vi "Launch Instrumentstudio.vi"(11 "error in (no error)":errorcluster) -> (15 "error out":errorcluster)   [LabVIEW 2021, in "Converter.lvlib"]
uses:
  Converter.lvlib
  Path Functions/Path Functions.lvlib
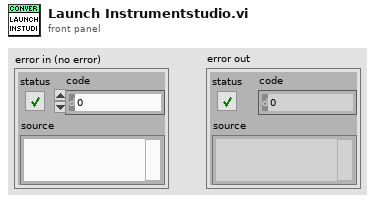
[diagram p1: front panel]
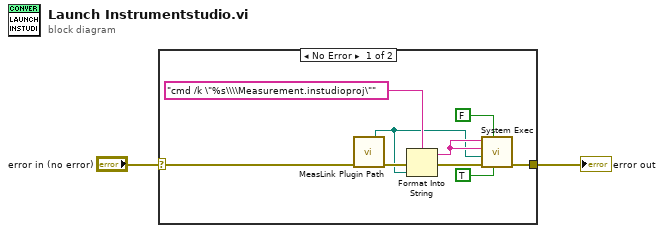
[diagram p0: block diagram]
diagram:
  n1 = case shown="No Error" "error in (no error)" {
    selector: "error in (no error)" -> [w9 w12]
    tunnel: [w3 w12] -> w1
    frame No Error {
      n2 = call "MeasLink Plugin Path.vi"("error in (no error)"=w9) -> ("Instrumentstudio Folder"=w5:path, "error out"=w10:errorcluster)  [unwired: 2 in, 11 out]
      n3 = Format Into String(format string="cmd /k \"%s\\\\Measurement.instudioproj\"", error in=w10, w5) -> (resulting string=w6:string, error out=w8:errorcluster)  [unwired: 1 in]
      n4 = call <vilib>:"System Exec.vi"("run minimized? (F)"=TRUE, "wait until completion? (T)"=FALSE, "error in (no error)"=w8, "working directory"=w5, "standard input"=w6, "command line"=w6) -> ("error out"=w3:errorcluster)  [unwired: 2 in, 3 out]
    }
    frame Error {
    }
  }
  "error out" <- w1
